vi "play aim set target.vi"(8 "Array":cluster{"Numeric":dbl, "Numeric 2":dbl}[](array[cluster]), 10 "BG Pic":picture) -> (1 "2D Picture":picture)   [LabVIEW 2014]
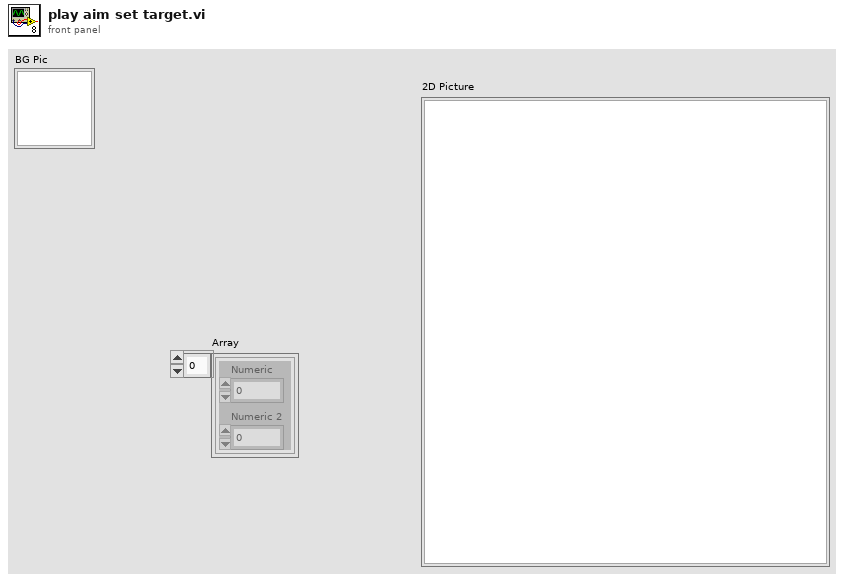
[diagram p1: front panel]
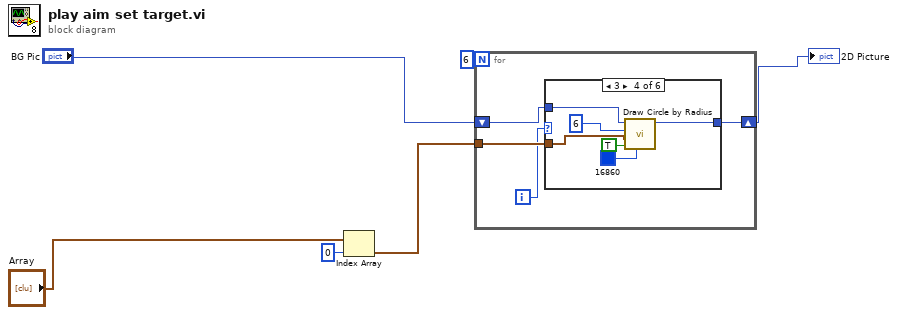
[diagram p0: block diagram]
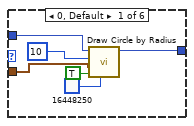
[diagram p2: hidden frame]
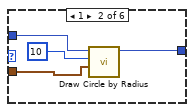
[diagram p3: hidden frame]
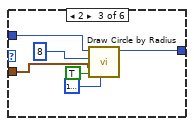
[diagram p4: hidden frame]
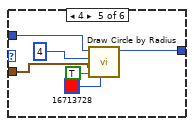
[diagram p5: hidden frame]
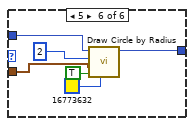
[diagram p6: hidden frame]
diagram:
  n1 = Index Array(array="Array", index=0) -> (element=w2:cluster{"Numeric":dbl, "Numeric 2":dbl})
  n2 = for {
    N: 6 -> [_]
    tunnel: w2 -> [w10]
    shift-right: [w9] -> w6
    shift-left: "BG Pic" -> [w7]
    i -> [w8]
    n3 = case shown="3" w8 {
      tunnel: w10 -> [w16 w20 w26 w32 w38 w44]
      tunnel: [w15 w19 w25 w31 w37 w43] -> w9
      tunnel: w7 -> [w11 w17 w21 w27 w33 w39]
      frame 0, Default {
        n4 = call <vilib>:"Draw Circle by Radius.vi"("color(black)"=u32 16448250, "fill?(F)"=TRUE, "pixel center"=w16, "radius"=i16 10, "picture"=w11) -> ("new picture"=w15:picture)  [unwired: 6 in]
      }
      frame 1 {
        n5 = call <vilib>:"Draw Circle by Radius.vi"("pixel center"=w20, "radius"=i16 10, "picture"=w17) -> ("new picture"=w19:picture)  [unwired: 8 in]
      }
      frame 2 {
        n6 = call <vilib>:"Draw Circle by Radius.vi"("color(black)"=u32 16777222, "fill?(F)"=TRUE, "pixel center"=w26, "radius"=i16 8, "picture"=w21) -> ("new picture"=w25:picture)  [unwired: 6 in]
      }
      frame 3 {
        n7 = call <vilib>:"Draw Circle by Radius.vi"("color(black)"=u32 16860, "fill?(F)"=TRUE, "pixel center"=w32, "radius"=i16 6, "picture"=w27) -> ("new picture"=w31:picture)  [unwired: 6 in]
      }
      frame 4 {
        n8 = call <vilib>:"Draw Circle by Radius.vi"("color(black)"=u32 16713728, "fill?(F)"=TRUE, "pixel center"=w38, "radius"=i16 4, "picture"=w33) -> ("new picture"=w37:picture)  [unwired: 6 in]
      }
      frame 5 {
        n9 = call <vilib>:"Draw Circle by Radius.vi"("color(black)"=u32 16773632, "fill?(F)"=TRUE, "pixel center"=w44, "radius"=i16 2, "picture"=w39) -> ("new picture"=w43:picture)  [unwired: 6 in]
      }
    }
  }
  "2D Picture" <- w6
